vi "fgv_ROI_Information.vi"(10 "ROI_Save_Enu":enum16{"Initialize", "write", "read"}(ring), 11 "ROI_Information_Cluster":T1 {"Norm. XYZ Coordinates"."ROI group ID" format="%#_6f"; "Norm. XYZ Coordinates"."Laser Power (%)" format="%#_6f"; "Norm. XYZ Coordinates"."Zoom" format="%#_6f"; "Norm. XYZ Coordinates"."Frame Size" format="%#_6f"; "Norm. XYZ Coordinates"."Number of lines" format="%#_6f"; "Norm. XYZ Coordinates"."Composite ID" format="%#_6f"; "Norm. XYZ Coordinates"."Angle (deg)" format="%#_6f"; "Norm. XYZ Coordinates"."ROI Time (ns)" format="%#_6f"; "Norm. XYZ Coordinates"."ROI ID" format="%#_6f"; "Norm. XYZ Coordinates"."Pixels in ROI" format="%#_6f"; "Norm. XYZ Coordinates"."ROI index" format="%#_6f"; "Norm. XYZ Coordinates"."Z stop" format="%#_6f"; "Norm. XYZ Coordinates"."Y stop" format="%#_6f"; "Norm. XYZ Coordinates"."X stop" format="%#_6f"; "Norm. XYZ Coordinates"."Z start" format="%#_6f"; "Norm. XYZ Coordinates"."X start" format="%#_6f"; "Norm. XYZ Coordinates"."Y start" format="%#_6f"; "XYZ Coordinates"."ROI group ID" format="%#_6f"; "XYZ Coordinates"."Laser Power (%)" format="%#_6f"; "XYZ Coordinates"."Zoom" format="%#_6f"; "XYZ Coordinates"."Frame Size" format="%#_6f"; "XYZ Coordinates"."Number of lines" format="%#_6f"; "XYZ Coordinates"."Composite ID" format="%#_6f"; "XYZ Coordinates"."Angle (deg)" format="%#_6f"; "XYZ Coordinates"."ROI Time (ns)" format="%#_6f"; "XYZ Coordinates"."ROI ID" format="%#_6f"; "XYZ Coordinates"."Pixels in ROI" format="%#_6f"; "XYZ Coordinates"."ROI index" format="%#_6f"; "XYZ Coordinates"."Z stop" format="%#_6f"; "XYZ Coordinates"."Y stop" format="%#_6f"; "XYZ Coordinates"."X stop" format="%#_6f"; "XYZ Coordinates"."Z start" format="%#_6f"; "XYZ Coordinates"."X start" format="%#_6f"; "XYZ Coordinates"."Y start" format="%#_6f"}) -> ()   [LabVIEW 2017]
uses:
  Typedefs/Controls/ROI_Information.ctl
  Visualisation/Functional Imaging Viewer/Typedefs/ROI parameters data type.ctl
panel:
  out "ROI_Information_Cluster":T1 {"Norm. XYZ Coordinates"."ROI group ID" format="%#_6f"; "Norm. XYZ Coordinates"."Laser Power (%)" format="%#_6f"; "Norm. XYZ Coordinates"."Zoom" format="%#_6f"; "Norm. XYZ Coordinates"."Frame Size" format="%#_6f"; "Norm. XYZ Coordinates"."Number of lines" format="%#_6f"; "Norm. XYZ Coordinates"."Composite ID" format="%#_6f"; "Norm. XYZ Coordinates"."Angle (deg)" format="%#_6f"; "Norm. XYZ Coordinates"."ROI Time (ns)" format="%#_6f"; "Norm. XYZ Coordinates"."ROI ID" format="%#_6f"; "Norm. XYZ Coordinates"."Pixels in ROI" format="%#_6f"; "Norm. XYZ Coordinates"."ROI index" format="%#_6f"; "Norm. XYZ Coordinates"."Z stop" format="%#_6f"; "Norm. XYZ Coordinates"."Y stop" format="%#_6f"; "Norm. XYZ Coordinates"."X stop" format="%#_6f"; "Norm. XYZ Coordinates"."Z start" format="%#_6f"; "Norm. XYZ Coordinates"."X start" format="%#_6f"; "Norm. XYZ Coordinates"."Y start" format="%#_6f"; "XYZ Coordinates"."ROI group ID" format="%#_6f"; "XYZ Coordinates"."Laser Power (%)" format="%#_6f"; "XYZ Coordinates"."Zoom" format="%#_6f"; "XYZ Coordinates"."Frame Size" format="%#_6f"; "XYZ Coordinates"."Number of lines" format="%#_6f"; "XYZ Coordinates"."Composite ID" format="%#_6f"; "XYZ Coordinates"."Angle (deg)" format="%#_6f"; "XYZ Coordinates"."ROI Time (ns)" format="%#_6f"; "XYZ Coordinates"."ROI ID" format="%#_6f"; "XYZ Coordinates"."Pixels in ROI" format="%#_6f"; "XYZ Coordinates"."ROI index" format="%#_6f"; "XYZ Coordinates"."Z stop" format="%#_6f"; "XYZ Coordinates"."Y stop" format="%#_6f"; "XYZ Coordinates"."X stop" format="%#_6f"; "XYZ Coordinates"."Z start" format="%#_6f"; "XYZ Coordinates"."X start" format="%#_6f"; "XYZ Coordinates"."Y start" format="%#_6f"}
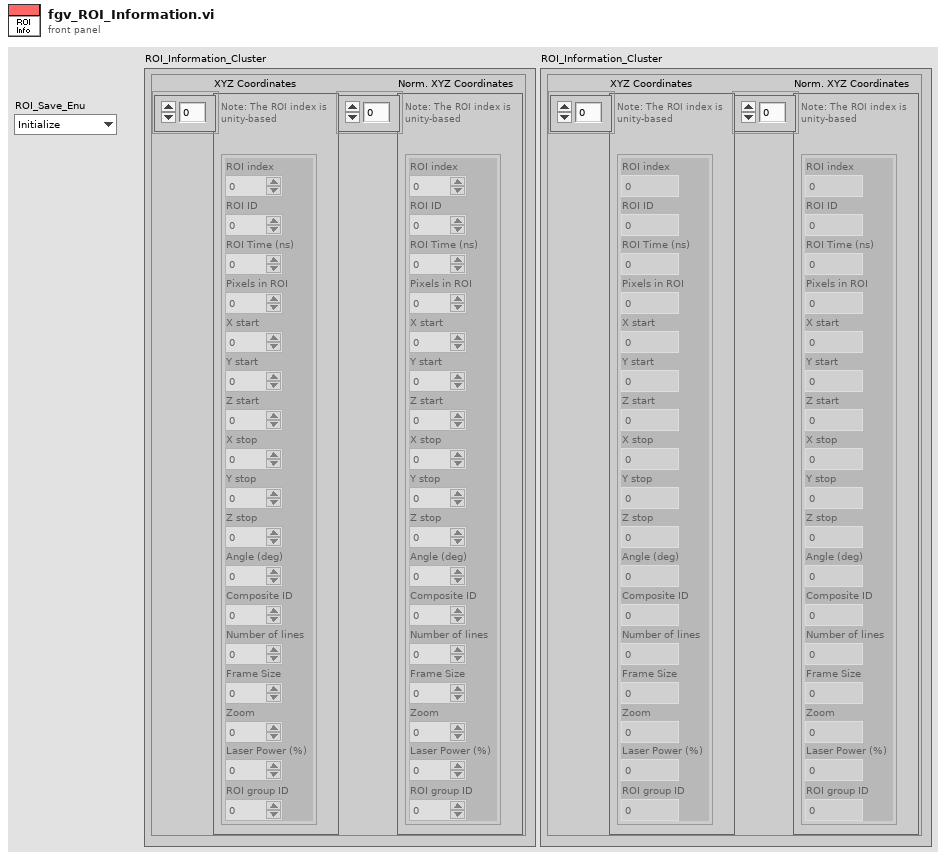
[diagram p1: front panel]
types:
  T1 = typedef "ROI_Information.ctl" = cluster{"XYZ Coordinates":T2[], "Norm. XYZ Coordinates":T2[]}
  T2 = typedef "ROI parameters data type.ctl" = cluster{"ROI index":dbl, "ROI ID":dbl, "ROI Time (ns)":dbl, "Pixels in ROI":dbl, "X start":dbl, "Y start":dbl, "Z start":dbl, "X stop":dbl, "Y stop":dbl, "Z stop":dbl, "Angle (deg)":dbl, "Composite ID":dbl, "Number of lines":dbl, "Frame Size":dbl, "Zoom":dbl, "Laser Power (%)":dbl, "ROI group ID":dbl}
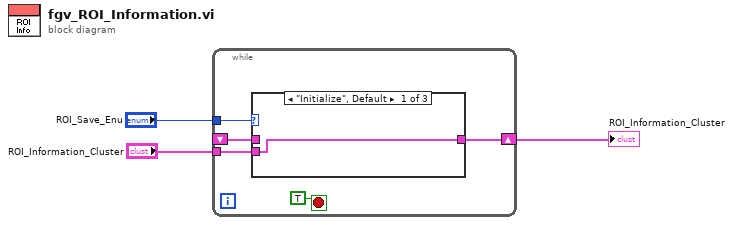
[diagram p0: block diagram]
diagram:
  n1 = while {
    tunnel: "ROI_Save_Enu" -> [w7]
    tunnel: "ROI_Information_Cluster" -> [w4]
    shift-right: [w6] -> w1
    shift-left: _ -> [w5]
    stop <- TRUE stop-if-true
    n2 = case shown="\"Initialize\", Default" w7 {
      tunnel: w5 -> [_ _ w11]
      tunnel: [w9 w10 w11] -> w6
      tunnel: w4 -> [w9 w10 _]
      frame "Initialize", Default {
      }
      frame "write" {
      }
      frame "read" {
      }
    }
  }
  "ROI_Information_Cluster" <- w1
